vi "AB_Engine_LinkerErrorVerboseShouldAnalyze.vi"(10 "viflags2":u32, 11 "type":T1) -> (2 "Should Analyze?":bool)   [LabVIEW 2020]
uses:
  <vilib>/Utility/lvfile.llb/LVFileType.ctl
  <vilib>/Utility/lvfile.llb/NI_FileType.lvlib
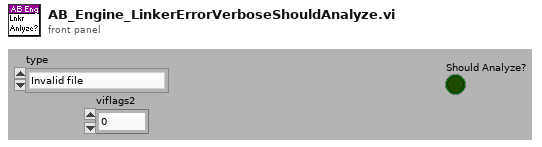
[diagram p1: front panel]
types:
  T1 = typedef "NI_FileType.lvlib/LVFileType.ctl" = enum32{"Invalid file", "Unknown type", "Instrument", "Control", "Polymorphic VI", "Project", "Library", "LVClass", "XControl", "XNode", "Shared library", ".NET assembly", "ActiveX interface", "CIN", "Run-time menu", "Palette menu", "Help file", "LLB", "XNode Edit Dependency", "Class Private Data Control", "Statechart", "MathScript .m file", "Ladder Diagram", "LVLibp", "XNode Build Dependency"}
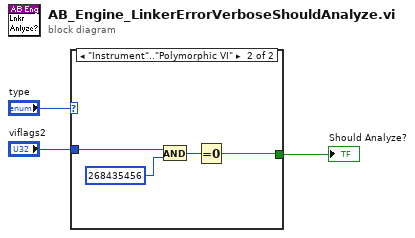
[diagram p0: block diagram]
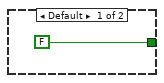
[diagram p2: hidden frame]
diagram:
  n1 = case shown="\"Instrument\"..\"Polymorphic VI\"" "type" {
    tunnel: [FALSE w5] -> w2
    tunnel: "viflags2" -> [_ w8]
    frame Default {
    }
    frame "Instrument".."Polymorphic VI" {
      n2 = And(x=w8, y=u32 268435456 ("viflags")) -> (x .and. y?=w6:u32)
      n3 = Equal To 0?(x=w6) -> (x = 0?=w5:bool)
    }
  }
  "Should Analyze?" <- w2
